vi "Convert Impedance.vi"(9 "Input Impedance (0 Ohm)":dbl, 11 "Discrete Value List":dbl[](array[numeric])) -> (1 "Output Impedance":dbl=50.0)   [LabVIEW 2012, in "Fluke 5080.lvlib"]
doc: "Converts the impendance value to the instrument acceptable level."
uses:
  <instrlib>/Fluke 5080/Fluke 5080.lvlib
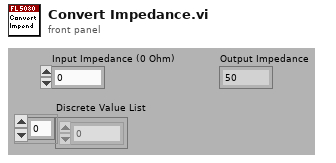
[diagram p1: front panel]
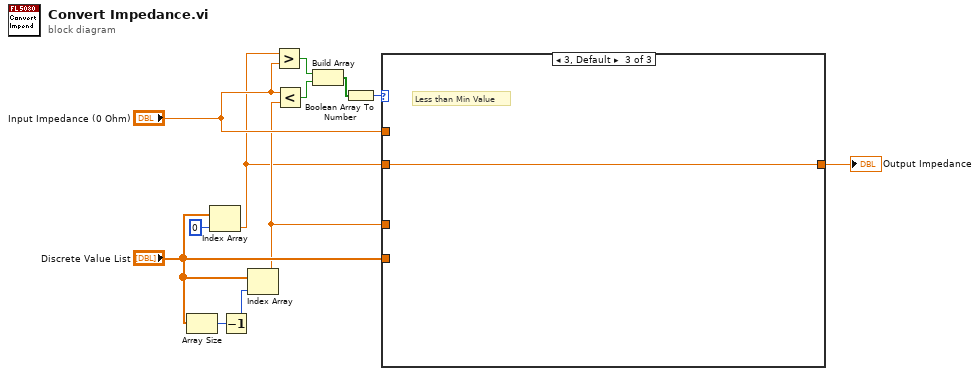
[diagram p0: block diagram]
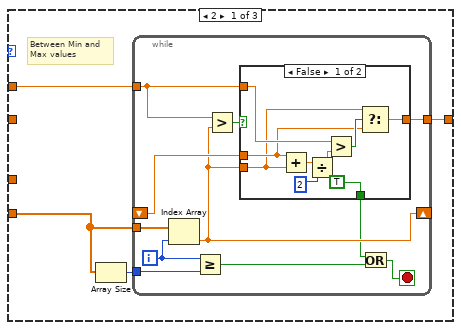
[diagram p2: hidden frame]
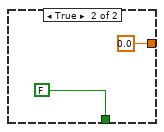
[diagram p3: hidden frame]
diagram:
  n1 = Array Size(array="Discrete Value List") -> (size(s)=w5:i32)
  n2 = Index Array(array="Discrete Value List", index=0) -> (element=w1:dbl)
  n3 = Decrement(x=w5) -> (x-1=w4:i32)
  n4 = Index Array(array="Discrete Value List", index=w4) -> (element=w2:dbl)
  n5 = Greater?(x=w1, y="Input Impedance (0 Ohm)") -> (0:w12:bool)
  n6 = Less?(x="Input Impedance (0 Ohm)", y=w2) -> (x < y?=w11:bool)
  n7 = Build Array(w12, w11) -> (w10:bool[])
  n8 = Boolean Array To Number(Boolean array=w10) -> (number=w9:u32)
  n9 = case shown="3, Default" w9 {
    tunnel: [w14 w39 w40] -> w8
    tunnel: "Input Impedance (0 Ohm)" -> [w15 _ _]
    tunnel: "Discrete Value List" -> [w13 _ _]
    tunnel: w2 -> [_ w39 _]
    tunnel: w1 -> [_ _ w40]
    frame 2 {
      # "Between Min and\nMax values"
      n10 = Array Size(array=w13) -> (size(s)=w16:i32)
      n11 = while {
        tunnel: w13 -> [w23]
        tunnel: w16 -> [w27]
        shift-right: [w21] -> _
        shift-left: _ -> [w22]
        tunnel: w15 -> [w17]
        tunnel: [w18] -> w14
        i -> [w24]
        stop <- w26 stop-if-true
        n12 = Index Array(array=w23, index=w24) -> (element=w21:dbl)
        n13 = Greater Or Equal?(x=w24, y=w27) -> (x >= y?=w25:bool)
        n14 = Greater?(x=w17, y=w21) -> (0:w20:bool)
        n15 = case shown="False" w20 {
          tunnel: w22 -> [w31 _]
          tunnel: w21 -> [w30 _]
          tunnel: [TRUE ("x") FALSE ("x")] -> w19
          tunnel: [w29 0.0 ("Output Impedance")] -> w18
          tunnel: w17 -> [w34 _]
          frame False {
            n16 = Add(x=w31, y=w30) -> (x+y=w36:dbl)
            n17 = Divide(x=w36, y=2) -> (x/y=w33:dbl)
            n18 = Greater?(x=w34, y=w33) -> (0:w32:bool)
            n19 = Select(t=w30, s=w32, f=w31) -> (s? t:f=w29:dbl)
          }
          frame True {
          }
        }
        n20 = Or(x=w19, y=w25) -> (x .or. y?=w26:bool)
      }
    }
    frame 0 {
      # "Greater than Max value"
    }
    frame 3, Default {
      # "Less than Min Value"
    }
  }
  "Output Impedance" <- w8
